vi "FPGA_Main.vi"() -> ()   [LabVIEW 2018]
uses:
  <vilib>/rvi/FXPMathLib/FxpDiv/subVIs/nifxpmath_Div_SimConfig.ctl
  <vilib>/rvi/FXPMathLib/FxpAtan2/subVIs/nifxpmath_Atan2_SimConfig.ctl
  <vilib>/rvi/FXPMathLib/FxpSinAndCos/subVIs/nifxpmath_SinAndCos_SimConfig.ctl
  <vilib>/rvi/Emulation/niFpgaGetClockAttributes.vi
  <vilib>/rvi/Emulation/niFpgaSctlEmulationGetInTimedLoop.vi
  <vilib>/rvi/Emulation/niFpgaEmulationReportErrorSimple.vi
  <vilib>/rvi/eio/common/nirviEmuTemplateMethod_errors.vi
  <vilib>/rvi/Emulation/niFpgaProcessEmulError.vi
  <vilib>/rvi/FXPMathLib/FxpDiv/simVIs/DllFxpDivTemp_sub.vi
  <vilib>/rvi/FXPMathLib/FxpAtan2/simVIs/DllFxpAtan2Temp_sub.vi
  <vilib>/rvi/FXPMathLib/FxpSinAndCos/simVIs/DllFxpSinAndCosTemp_sub.vi
  <vilib>/rvi/interface/RandomDataEmulation/nirviRandomDataMultiElementFPGAFIFO.vi
  <instcachedir>/0/nirviRandomDataMultiElementFPGAFIFO_6740B454F3C245F78F76ED91F73FD8DB.lvgen/nirviRandomDataMultiElementFPGAFIFO_6740B454F3C245F78F76ED91F73FD8DB_007.vi
  <vilib>/rvi/interface/RandomDataEmulation/niFpgaRandomDataHandleErrors.vi
  <vilib>/rvi/Emulation/niFpgaCriticalErrorInLSC.vi
  <vilib>/eio/EIONode/EIONode.xnode
  <vilib>/rvi/FXPMathLib/FxpMul/XNode/nifxpmath_Multiplier.xnode
  <vilib>/rvi/Analysis/measure/butterworth/XNode/niFpgaButterworthFilter.xnode
  <vilib>/rvi/FXPMathLib/FxpSub/XNode/nifxpmath_Sub.xnode
  <vilib>/rvi/FXPMathLib/FxpDiv/XNode/nifxpmath_Div.xnode
  <vilib>/rvi/Analysis/measure/notch/XNode/niFpgaNotchFilter.xnode
  <vilib>/rvi/FXPMathLib/FxpAtan2/XNode/nifxpmath_Atan2.xnode
  <vilib>/rvi/FXPMathLib/FxpAdd/XNode/nifxpmath_Add.xnode
  <vilib>/rvi/FXPMathLib/FxpSinAndCos/XNode/nifxpmath_SinAndCos.xnode
  <vilib>/rvi/DataTransferAndStorage/Container/XNode/niFpgaContainer.xnode
  <vilib>/rvi/interface/RandomDataEmulation/nirviRandomDataFpgaMultiElementTemplate.vi
  <vilib>/rvi/FXPMathLib/sim/FxpSim.dll
panel:
  in  "phase_correction":fxp<+/-,16,2>[](array[numeric])=[0.0, 0.0]
  in  "Filter coeffs":i32[](array[numeric])=[0, 0, 0, 0, 0, 0, 0, 0, 0, 0, 0, 0]
  in  "idx scope":u8=25
  in  "gain":fxp<+,18,6>=1.0
  in  "base freqs":fxp<+,17,17>[](array[numeric])=[0.0, 0.0]
  in  "idx pick":u8=25
  in  "reset":bool
  in  "I gain":fxp<+,20,6>
  in  "P gain":fxp<+,14,14>=700.0
  # "FPGA Main"
  # "Shared variables for interaction with RT- and PC-Main"
  # "Enable only in simulation mode!"
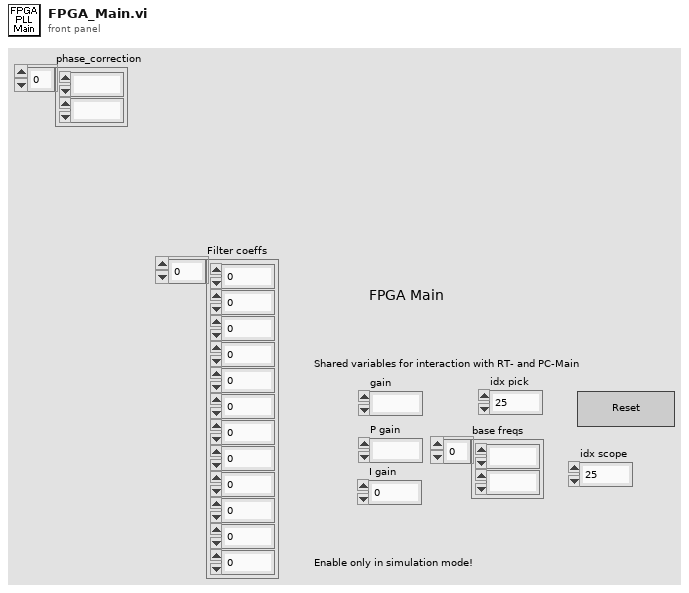
[diagram p1: front panel]
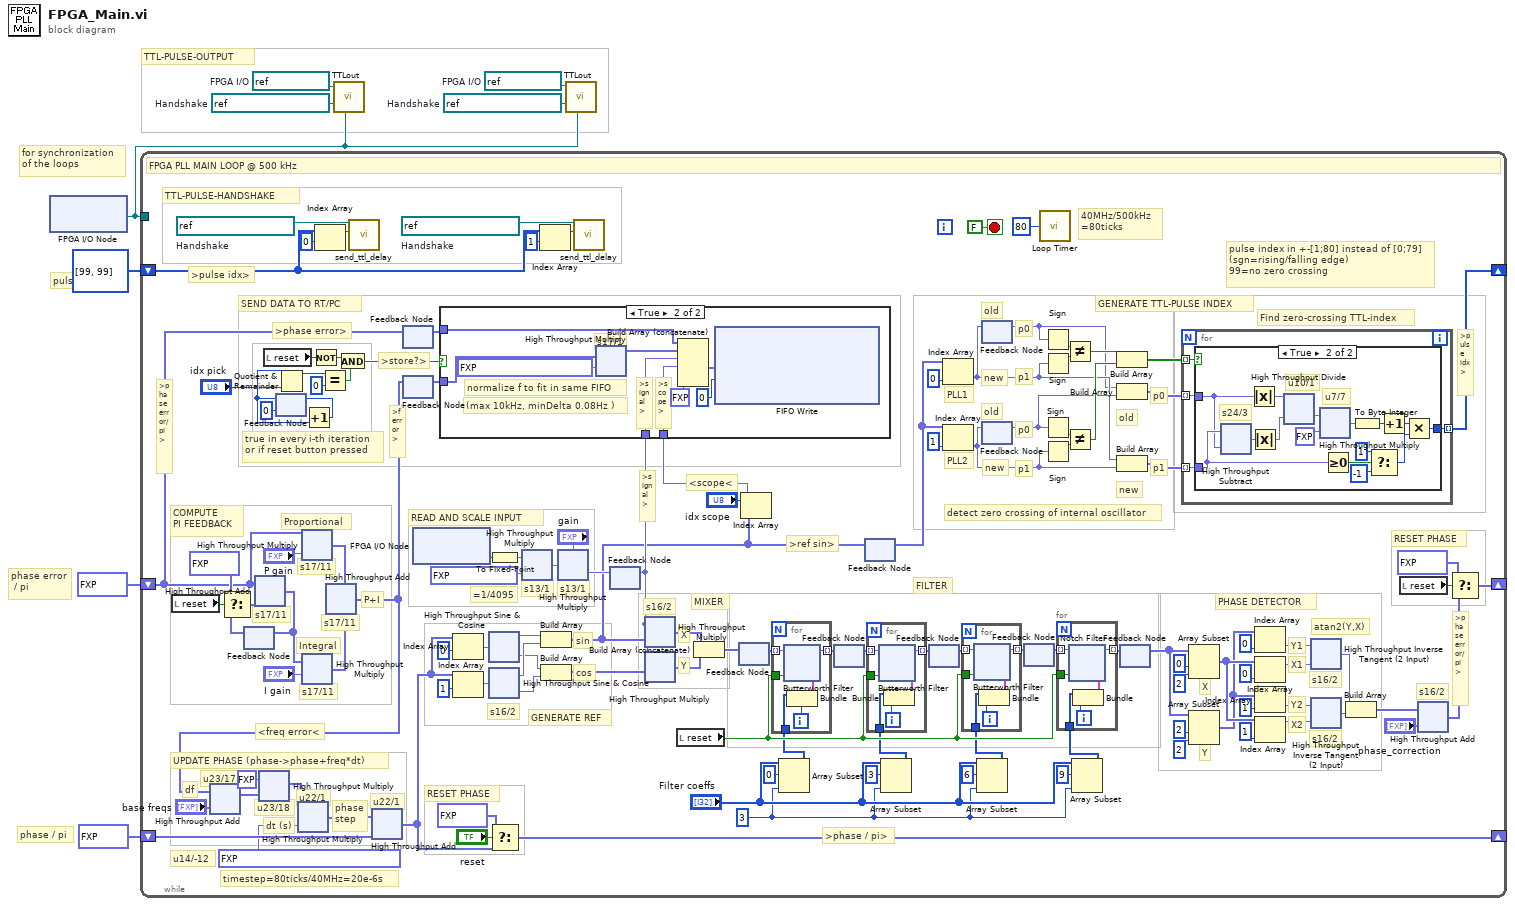
[diagram p0: block diagram]
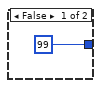
[diagram p2: hidden frame]
diagram:
  w2 = refnum<k21> "TTL-out2"  # FPGA I/O
  w3 = refnum<k21> "TTL_Handshake2"  # Handshake
  w5 = refnum<k21> "TTL-out1"  # FPGA I/O
  w4 = refnum<k21> "TTL_Handshake1"  # Handshake
  # "TTL-PULSE-OUTPUT"
  # "for synchronization\nof the loops"
  # "pulse idx"
  # "phase error\n / pi"
  # "phase / pi"
  n1 = xnode "FPGA I/O Node"() -> ("FPGA I/O Out"=w1:refnum<k21>)  [unwired: 1 in, 1 out]
  n2 = while {
    shift-right: [w132] -> _
    shift-left: fxp<+/-,1,0>[] [0.0, 0.0] ("t") -> [w131]
    shift-right: [w130] -> _
    shift-left: fxp<+/-,16,2>[] [0.0, 0.0] ("t") -> [w73]
    shift-right: [w54] -> _
    shift-left: i8[] [99, 99] ("idx array") -> [w71]
    tunnel: w1 -> [_]
    stop <- FALSE stop-if-true
    w16 = 3 ("index")
    w123 = refnum<k21> "TTL_Handshake2"  # Handshake
    w128 = refnum<k21> "TTL_Handshake1"  # Handshake
    # "s16/2"
    # ">phase error/pi>"
    # "Y"
    # "X"
    # "FILTER"
    # "MIXER"
    # "<scope<"
    # ">pulse idx>"
    # ">pulse idx>"
    # ">store?>"
    # ">phase error>"
    # ">signal>"
    # "X2"
    # "Y2"
    # "X1"
    # "Y1"
    # "40MHz/500kHz\n=80ticks"
    # "COMPUTE\nPI FEEDBACK"
    # "GENERATE TTL-PULSE INDEX"
    # "pulse index in +-[1;80] instead of [0;79]\n(sgn=rising/falling edge)\n99=no zero crossing"
    # "Find zero-crossing TTL-index"
    # "detect zero crossing of internal oscillator"
    # "s16/2"
    # "PHASE DETECTOR"
    # ">ref sin>"
    # "new"
    # "old"
    # "p1"
    # "p0"
    # "PLL2"
    # "PLL1"
    # "p1"
    # "p0"
    # "new"
    # "old"
    # "p1"
    # "p0"
    # "new"
    # "old"
    # "s16/2"
    # "s16/2"
    # "atan2(Y,X)"
    # "dt (s)"
    # "u23/17"
    # "u23/18"
    # "u22/1"
    # "u22/1"
    # "df"
    # "UPDATE PHASE (phase->phase+freq*dt)"
    # "phase\nstep"
    # "s17/11"
    # "s17/11"
    # "s17/11"
    # "s17/11"
    # "P+I"
    # "Integral"
    # "Proportional"
    # "u14/-12"
    # "timestep=80ticks/40MHz=20e-6s"
    # "Y"
    # "X"
    # "s13/1"
    # "READ AND SCALE INPUT"
    # "true in every i-th iteration \nor if reset button pressed"
    # "SEND DATA TO RT/PC"
    # ">phase error/pi>"
    # "GENERATE REF"
    # "cos"
    # "sin"
    # "<freq error<"
    # "s16/2"
    # "s13/1"
    # "=1/4095"
    # "RESET PHASE"
    # ">f error>"
    # "RESET PHASE"
    # ">phase / pi>"
    # "TTL-PULSE-HANDSHAKE"
    # "FPGA PLL MAIN LOOP @ 500 kHz"
    n3 = local read "reset"() -> (w83:bool)
    n4 = feedback #1() -> (w84:fxp<+/-,17,11>[])  [unwired: 1 in]
    n5 = Select(t=fxp<+/-,16,10>[] [0.0, 0.0], s=w83, f=w84) -> (s? t:f=w72:fxp<+/-,17,11>[])
    n6 = xnode ("High Throughput Add")("x"=w73, "y"=w72) -> ("x+y"=w74:fxp<+/-,17,11>[])
    n7 = feedback-in #1(w74) -> ()
    n8 = local read "reset"() -> (w114:bool)
    n9 = feedback #2(i16 0) -> (w113:i16)
    n10 = Quotient & Remainder(x=w113, y="idx pick") -> (x-y*floor(x/y)=w119:i16)  [unwired: 1 out]
    n11 = xnode ("High Throughput Multiply")("x"=w73, "y"="P gain") -> ("x*y"=w87:fxp<+/-,17,11>[])
    n12 = xnode ("High Throughput Multiply")("x"=w74, "y"="I gain") -> ("x*y"=w88:fxp<+/-,17,11>[])
    n13 = Increment(x=w113) -> (x+1=w112:i16)
    n14 = feedback-in #2(w112) -> ()
    n15 = Not(x=w114) -> (.not. x?=w115:bool)
    n16 = Index Array(array=w71, index=0) -> (element=w126:i8)
    n17 = Equal?(x=w119, y=i16 0) -> (x = y?=w111:bool)
    n18 = xnode ("High Throughput Add")("x"=w87, "y"=w88) -> ("x+y"=w38:fxp<+/-,17,11>[])
    n19 = xnode ("High Throughput Add")("x"=w38, "y"="base freqs") -> ("x+y"=w79:fxp<+,23,17>[])
    n20 = xnode ("High Throughput Multiply")("x"=fxp<+,2,2> 2.0 ("y"), "y"=w79) -> ("x*y"=w81:fxp<+,23,18>[])
    n21 = xnode ("High Throughput Multiply")("x"=w81, "y"=fxp<+,14,-18> 2.00001522898674e-06) -> ("x*y"=w80:fxp<+,22,1>[])
    n22 = And(x=w115, y=w111) -> (x .and. y?=w116:bool)
    n23 = call "send_ttl_delay.vi"("delay index"=w126, "Handshake"=w128) -> ()  [unwired: 10 in]
    n24 = xnode ("High Throughput Add")("x"=w80, "y"=w131) -> ("x+y"=w55:fxp<+,22,1>[])
    n25 = feedback #3() -> (w97:fxp<+/-,16,2>[])  [unwired: 1 in]
    n26 = feedback-in #3(w73) -> ()
    n27 = feedback #4() -> (w98:fxp<+/-,17,11>[])  [unwired: 1 in]
    n28 = feedback-in #4(w38) -> ()
    n29 = xnode "FPGA I/O Node"() -> ("REF-in"=w96:i16)  [unwired: 1 in, 1 out]
    n30 = Index Array(array=w55, index=0) -> (element=w105:fxp<+,22,1>)
    n31 = Index Array(array=w55, index=1) -> (element=w104:fxp<+,22,1>)
    n32 = xnode "High Throughput Sine & Cosine"("x (pi)"=w105) -> ("sin(x)"=w103:fxp<+/-,16,2>, "cos(x)"=w101:fxp<+/-,16,2>)
    n33 = xnode "High Throughput Sine & Cosine"("x (pi)"=w104) -> ("sin(x)"=w102:fxp<+/-,16,2>, "cos(x)"=w100:fxp<+/-,16,2>)
    n34 = To Fixed-Point(number=w96) -> (fixed-point=w122:fxp<+/-,12,12>)  [unwired: 1 in]
    n35 = Select(t=fxp<+/-,1,0>[] [0.0, 0.0], s="reset", f=w55) -> (s? t:f=w132:fxp<+/-,23,2>[])
    n36 = xnode ("High Throughput Multiply")("x"=w122, "y"=fxp<+,12,0> 0.000244140625) -> ("x*y"=w92:fxp<+/-,13,1>)
    n37 = Index Array(array=w71, index=1) -> (element=w125:i8)
    n38 = Build Array(w103, w102) -> (w23:fxp<+/-,16,2>[])
    n39 = Build Array(w101, w100) -> (w99:fxp<+/-,16,2>[])
    n40 = xnode ("High Throughput Multiply")("x"="gain", "y"=w92) -> ("x*y"=w91:fxp<+/-,13,1>)
    n41 = call "send_ttl_delay.vi"("delay index"=w125, "Handshake"=w123) -> ()  [unwired: 10 in]
    n42 = feedback #5() -> (w95:fxp<+/-,13,1>)  [unwired: 1 in]
    n43 = feedback-in #5(w91) -> ()
    n44 = xnode ("High Throughput Multiply")("x"=w95, "y"=w23) -> ("x*y"=w47:fxp<+/-,16,2>[])
    n45 = xnode ("High Throughput Multiply")("x"=w95, "y"=w99) -> ("x*y"=w46:fxp<+/-,16,2>[])
    n46 = local read "reset"() -> (w27:bool)
    n47 = Build Array (concatenate)(w47, w46) -> (w45:fxp<+/-,16,2>[])
    n48 = feedback #6() -> (w24:fxp<+/-,16,2>[])  [unwired: 1 in]
    n49 = feedback-in #6(w45) -> ()
    n50 = Index Array(array=w23, index="idx scope") -> (element=w52:fxp<+/-,16,2>)
    n51 = case shown="True" w116 {
      tunnel: w97 -> [_ w360]
      tunnel: w95 -> [_ w359]
      tunnel: w98 -> [_ w358]
      tunnel: w52 -> [_ w357]
      frame False {
      }
      frame True {
        w356 = fxp<+,12,0> 0.0 ("x*y")
        # ">scope>"
        # "(max 10kHz, minDelta 0.08Hz )"
        # ">signal>"
        # "normalize f to fit in same FIFO"
        # "s17/1"
        # "send data until queue is full"
        n52 = xnode ("High Throughput Multiply")("x"=w358, "y"=fxp<+/-,22,1> 0.00010013580322265625) -> ("x*y"=w361:fxp<+/-,17,1>[])
        n53 = Build Array (concatenate)(w360, w361, w359, w357, w356, w356) -> (w362:fxp<+/-,18,2>[])
        n54 = xnode ("FIFO Write")("Element"=w362, "Timeout"=i16 0) -> ()  [unwired: 1 in, 2 out]
      }
    }
    n55 = Array Subset(array="Filter coeffs", index=0, length=w16) -> (w15:i32[])
    n56 = for {
      tunnel: w27 -> [w183]
      tunnel: w24 -> [w182] mode=indexing
      tunnel: [w181] -> w32 mode=indexing
      tunnel: w15 -> [w180]
      i -> [w178]
      n57 = Bundle(w180, w178) -> (w179:cluster{i32[], i32})  [unwired: 1 in]
      n58 = xnode "Butterworth Filter"("input data"=w182, "reset"=w183, "configuration"=w179) -> ("output data"=w181:fxp<+/-,16,2>)  [unwired: 1 out]
    }
    n59 = feedback #7() -> (w33:fxp<+/-,16,2>[])  [unwired: 1 in]
    n60 = feedback-in #7(w32) -> ()
    n61 = feedback #8() -> (w22:fxp<+/-,16,2>[])  [unwired: 1 in]
    n62 = feedback-in #8(w23) -> ()
    n63 = Array Subset(array="Filter coeffs", index=3, length=w16) -> (w14:i32[])
    n64 = for {
      tunnel: w27 -> [w168]
      tunnel: w33 -> [w167] mode=indexing
      tunnel: [w166] -> w28 mode=indexing
      tunnel: w14 -> [w163]
      i -> [w165]
      n65 = Bundle(w163, w165) -> (w164:cluster{i32[], i32})  [unwired: 1 in]
      n66 = xnode "Butterworth Filter"("input data"=w167, "reset"=w168, "configuration"=w164) -> ("output data"=w166:fxp<+/-,16,2>)  [unwired: 1 out]
    }
    n67 = feedback #9() -> (w29:fxp<+/-,16,2>[])  [unwired: 1 in]
    n68 = feedback-in #9(w28) -> ()
    n69 = Index Array(array=w22, index=0) -> (element=w64:fxp<+/-,16,2>)
    n70 = Index Array(array=w22, index=1) -> (element=w69:fxp<+/-,16,2>)
    n71 = Array Subset(array="Filter coeffs", index=6, length=w16) -> (w13:i32[])
    n72 = for {
      tunnel: w27 -> [w151]
      tunnel: w29 -> [w153] mode=indexing
      tunnel: [w152] -> w30 mode=indexing
      tunnel: w13 -> [w148]
      i -> [w150]
      n73 = Bundle(w148, w150) -> (w149:cluster{i32[], i32})  [unwired: 1 in]
      n74 = xnode "Butterworth Filter"("input data"=w153, "reset"=w151, "configuration"=w149) -> ("output data"=w152:fxp<+/-,16,2>)  [unwired: 1 out]
    }
    n75 = feedback #10() -> (w63:fxp<+/-,16,2>)  [unwired: 1 in]
    n76 = feedback-in #10(w64) -> ()
    n77 = feedback #11() -> (w68:fxp<+/-,16,2>)  [unwired: 1 in]
    n78 = feedback-in #11(w69) -> ()
    n79 = feedback #12() -> (w31:fxp<+/-,16,2>[])  [unwired: 1 in]
    n80 = feedback-in #12(w30) -> ()
    n81 = call "Loop Timer"("Count(Ticks)"=u32 80) -> ()  [unwired: 1 out]
    n82 = Sign(1:w63) -> (0:w61:fxp<+/-,2,2>)
    n83 = Sign(1:w64) -> (0:w62:fxp<+/-,2,2>)
    n84 = Sign(1:w68) -> (0:w67:fxp<+/-,2,2>)
    n85 = Sign(1:w69) -> (0:w66:fxp<+/-,2,2>)
    n86 = Not Equal?(x=w61, y=w62) -> (x != y?=w65:bool)
    n87 = Not Equal?(x=w67, y=w66) -> (x != y?=w70:bool)
    n88 = Array Subset(array="Filter coeffs", index=9, length=w16) -> (w12:i32[])
    n89 = for {
      tunnel: w27 -> [w136]
      tunnel: w31 -> [w138] mode=indexing
      tunnel: [w137] -> w26 mode=indexing
      tunnel: w12 -> [w133]
      i -> [w135]
      n90 = Bundle(w133, w135) -> (w134:cluster{i32[], i32})  [unwired: 1 in]
      n91 = xnode "Notch Filter"("input data"=w138, "reset"=w136, "configuration"=w134) -> ("output data"=w137:fxp<+/-,16,2>)  [unwired: 1 out]
    }
    n92 = Build Array(w65, w70) -> (w59:bool[])
    n93 = Build Array(w63, w68) -> (w58:fxp<+/-,16,2>[])
    n94 = Build Array(w64, w69) -> (w60:fxp<+/-,16,2>[])
    n95 = feedback #13() -> (w25:fxp<+/-,16,2>[])  [unwired: 1 in]
    n96 = feedback-in #13(w26) -> ()
    n97 = for {
      tunnel: w58 -> [w196] mode=indexing
      tunnel: w59 -> [w195] mode=indexing
      tunnel: w60 -> [w194] mode=indexing
      tunnel: [w193] -> w54 mode=indexing
      n98 = case shown="True" w195 {
        tunnel: w196 -> [_ w198]
        tunnel: w194 -> [_ w206]
        tunnel: [i8 99 w208] -> w193
        frame False {
        }
        frame True {
          # "u7/7"
          # "u10/1"
          # "s24/3"
          n99 = xnode "High Throughput Subtract"("x"=w206, "y"=w198) -> ("x-y"=w201:fxp<+/-,24,3>)
          n100 = Absolute Value(x=w198) -> (abs(x)=w199:fxp<+,16,2>)
          n101 = Absolute Value(x=w201) -> (abs(x)=w200:fxp<+,24,3>)
          n102 = xnode "High Throughput Divide"("x"=w199, "y"=w200) -> ("x/y"=w211:fxp<+,10,1>)
          n103 = xnode ("High Throughput Multiply")("x"=w211, "y"=fxp<+,7,7> 79.0 ("x")) -> ("x*y"=w212:fxp<+,7,7>)
          n104 = Greater Or Equal To 0?(x=w206) -> (x >= 0?=w207:bool)
          n105 = To Byte Integer(number=w212) -> (8bit integer=w202:i8)
          n106 = Select(t=i8 1 ("index"), s=w207, f=i8 -1 ("index")) -> (s? t:f=w203:i8)
          n107 = Increment(x=w202) -> (x+1=w209:i8)
          n108 = Multiply(x=w209, y=w203) -> (x*y=w208:i8)
        }
      }
    }
    n109 = Array Subset(array=w25, index=0 ("length"), length=2) -> (w40:fxp<+/-,16,2>[])
    n110 = Array Subset(array=w25, index=2 ("length"), length=2) -> (w39:fxp<+/-,16,2>[])
    n111 = Index Array(array=w39, index=0) -> (element=w37:fxp<+/-,16,2>)
    n112 = Index Array(array=w40, index=0) -> (element=w36:fxp<+/-,16,2>)
    n113 = Index Array(array=w39, index=1) -> (element=w35:fxp<+/-,16,2>)
    n114 = Index Array(array=w40, index=1) -> (element=w34:fxp<+/-,16,2>)
    n115 = xnode "High Throughput Inverse Tangent (2 Input)"("y"=w37, "x"=w36) -> ("atan2(y,x) (pi)"=w76:fxp<+/-,16,2>)
    n116 = xnode "High Throughput Inverse Tangent (2 Input)"("y"=w35, "x"=w34) -> ("atan2(y,x) (pi)"=w77:fxp<+/-,16,2>)
    n117 = Build Array(w76, w77) -> (w11:fxp<+/-,16,2>[])
    n118 = local read "reset"() -> (w120:bool)
    n119 = xnode ("High Throughput Add")("x"=w11, "y"="phase_correction") -> ("x+y"=w9:fxp<+/-,16,2>[])
    n120 = Select(t=fxp<+/-,1,0>[] [0.0, 0.0], s=w120, f=w9) -> (s? t:f=w130:fxp<+/-,16,2>[])
  }
  n121 = call "TTLout.vi"("synch_signal"=w1, "Handshake"=w4, "FPGA I/O"=w5) -> ()  [unwired: 9 in]
  n122 = call "TTLout.vi"("synch_signal"=w1, "Handshake"=w3, "FPGA I/O"=w2) -> ()  [unwired: 9 in]
